vi "Read TDMS Wavenames.vi"(8 "error in (no error)":errorcluster, 10 "path":path, 11 "LVtoITX in":refnum<class "LVtoITX.lvclass">) -> (0 "error out":errorcluster, 2 "Wavenames":string[](array[string]), 3 "LVtoITX out":refnum<class "LVtoITX.lvclass">)   [LabVIEW 2016, in "LVtoITX.lvclass"]
uses:
  LVtoITX.lvclass
  LVtoITX.lvclass/LVtoITX.ctl
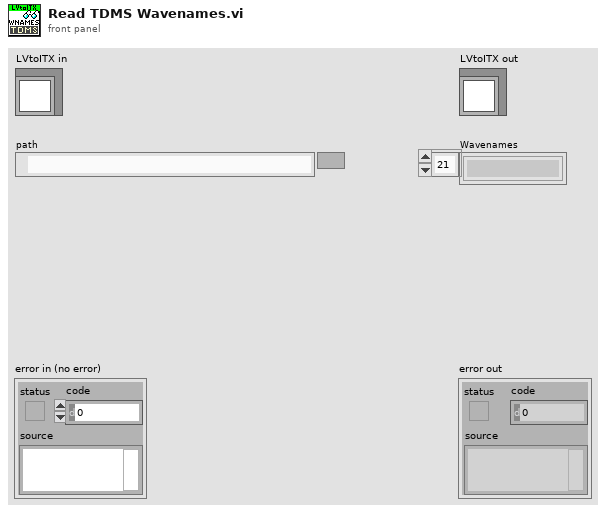
[diagram p1: front panel]
types:
  T1 = enum16{"open", "open or create", "create or replace", "create", "open (read-only)"}
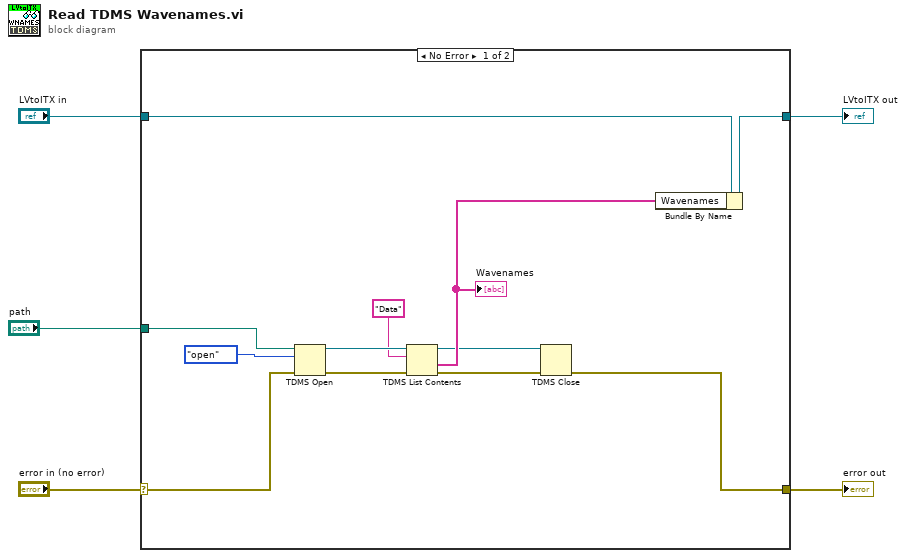
[diagram p0: block diagram]
diagram:
  n1 = case shown="No Error" "error in (no error)" {
    selector: "error in (no error)" -> [w6 w18]
    tunnel: [w12 w18] -> w2
    tunnel: [w16 w19] -> w3
    tunnel: "LVtoITX in" -> [w17 w19]
    tunnel: "path" -> [w10 _]
    frame No Error {
      n2 = TDMS Open(8:w6, 10:T1."open" ("operation (0:open)"), 11:w10) -> (0:w13:errorcluster, 3:w14:refnum<k34>)  [unwired: 4 in]
      n3 = TDMS List Contents(4:w13, 6:"Data" ("group name"), 7:w14) -> (0:w8:errorcluster, 1:w9:string[], 3:w7:refnum<k34>)  [unwired: 1 out]
      "Wavenames" <- w9
      n4 = TDMS Close(8:w8, 11:w7) -> (0:w12:errorcluster)  [unwired: 1 out]
      n5 = Bundle By Name(cluster=w17, "Wavenames"=w9) -> (w16:refnum<class "LVtoITX.lvclass">)
    }
    frame Error {
    }
  }
  "error out" <- w2
  "LVtoITX out" <- w3
